vi "Plot Counter.vi"(9 "y in":dbl, 11 "Numeric":dbl) -> (2 "y out":dbl, 3 "Boolean out":bool)   [LabVIEW 2019]
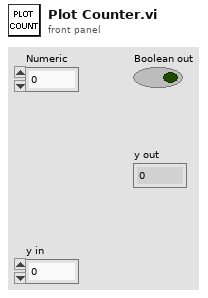
[diagram p1: front panel]
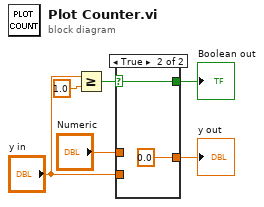
[diagram p0: block diagram]
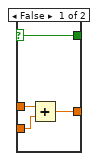
[diagram p2: hidden frame]
diagram:
  n1 = Greater Or Equal?(x="y in", y=1.0) -> (x >= y?=w2:bool)
  n2 = case shown="True" w2 {
    selector: w2 -> [w7 w11]
    tunnel: [w7 w11] -> w4
    tunnel: "Numeric" -> [w10 _]
    tunnel: "y in" -> [w9 _]
    tunnel: [w8 0.0 ("y")] -> w3
    frame False {
      n3 = Add(x=w10, y=w9) -> (x+y=w8:dbl)
    }
    frame True {
    }
  }
  "Boolean out" <- w4
  "y out" <- w3
